vi "Initialise.vi"(8 "error in (no error)":errorcluster, 10 "Message in":refnum<class "InitialiseMessage.lvclass">, 11 "Thorcam in":refnum<class "Thorcam.lvclass">) -> (0 "error out":errorcluster, 3 "Thorcam out":refnum<class "Thorcam.lvclass">)   [LabVIEW 2012, in "Thorcam.lvclass"]
doc: "This method is called when an initialise message is received. It mainly initialises the RabbitMQ connectivity. \n\nOverride this method when your component needs special initialisation (e.g. of software or hardware resources). In that case, don't forget to call the parent for proper implementation. If your component owns subcomponents, they count as resources, so you have to initialise them by calling their own initialise functions"
uses:
  Thorcam.lvclass
  <vilib>/Distrio/Murmex/InitialiseMessage/InitialiseMessage.lvclass
  <vilib>/Distrio/Murmex/Murmex/Murmex.lvclass
  Thorcam.lvclass/Thorcam.ctl
panel:
  # "This method is called when the INTIALISE\ntrigger is sent. \n\nOverride this method when your component needs to\nrespond to this trigger. \n\nCall parent for proper implementation"
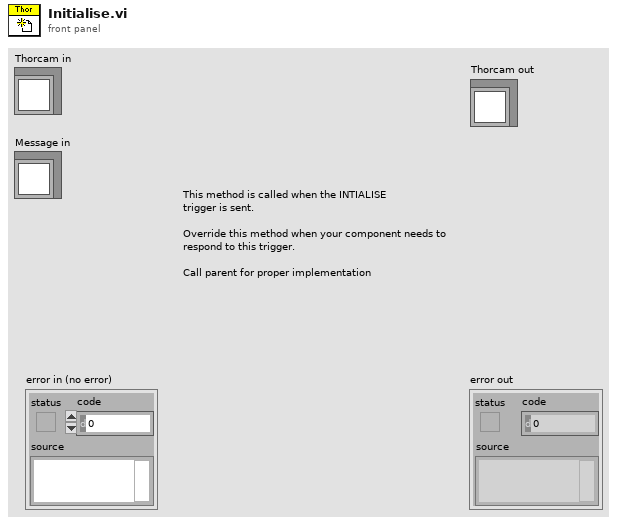
[diagram p1: front panel]
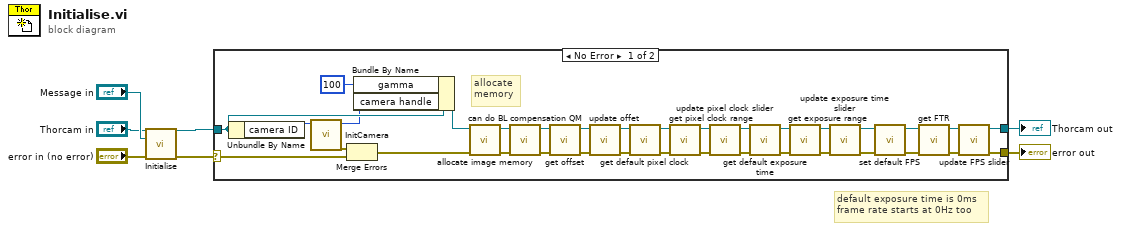
[diagram p0: block diagram]
diagram:
  # "default exposure time is 0ms\nframe rate starts at 0Hz too"
  n1 = call-parent "Initialise.vi"("error in (no error)"="error in (no error)", "Message in"="Message in", "Murmex in"="Thorcam in") -> ("error out"=w4:errorcluster, "Murmex out"=w3:refnum<class "Thorcam.lvclass">)  [unwired: 7 in]
  n2 = case shown="No Error" w4 {
    selector: w4 -> [w41 w42]
    tunnel: w3 -> [w38 w43]
    tunnel: [w27 w42] -> w2
    tunnel: [w28 w43] -> w1
    frame No Error {
      # "allocate\nmemory"
      n3 = Unbundle By Name(w38) -> ("camera ID"=w39:u32)
      n4 = call <instrlib>:"InitCamera.vi"("Camera ID"=w39) -> ("error out"=w40:errorcluster, "Camera Handle Out"=w37:u32)  [unwired: 9 in]
      n5 = Merge Errors(w40, w41) -> (w36:errorcluster)
      n6 = Bundle By Name(cluster=w38, "gamma"=100 ("settings.image.gamma"), "camera handle"=w37) -> (w35:refnum<class "Thorcam.lvclass">)
      n7 = call-dynamic "allocate image memory.vi"("error in (no error)"=w36, "Thorcam in"=w35) -> ("error out"=w34:errorcluster, "Thorcam out"=w33:refnum<class "Thorcam.lvclass">)  [unwired: 8 in]
      n8 = call-dynamic "can do BL compensation QM"("error in (no error)"=w34, "Thorcam in"=w33) -> ("error out"=w31:errorcluster, "Thorcam out"=w32:refnum<class "Thorcam.lvclass">)  [unwired: 8 in]
      n9 = call-dynamic "get offset.vi"("error in (no error)"=w31, "Thorcam in"=w32) -> ("error out"=w30:errorcluster, "Thorcam out"=w29:refnum<class "Thorcam.lvclass">)  [unwired: 8 in]
      n10 = call-dynamic "update offet.vi"("error in (no error)"=w30, "Thorcam in"=w29) -> ("error out"=w15:errorcluster, "Thorcam out"=w16:refnum<class "Thorcam.lvclass">)  [unwired: 8 in]
      n11 = call-dynamic "get default pixel clock.vi"("error in (no error)"=w15, "Thorcam in"=w16) -> ("error out"=w18:errorcluster, "Thorcam out"=w22:refnum<class "Thorcam.lvclass">)  [unwired: 7 in, 1 out]
      n12 = call-dynamic "get pixel clock range.vi"("error in (no error)"=w18, "Thorcam in"=w22) -> ("error out"=w17:errorcluster, "Thorcam out"=w21:refnum<class "Thorcam.lvclass">)  [unwired: 8 in]
      n13 = call-dynamic "update pixel clock slider.vi"("error in (no error)"=w17, "Thorcam in"=w21) -> ("error out"=w13:errorcluster, "Thorcam out"=w14:refnum<class "Thorcam.lvclass">)  [unwired: 8 in]
      n14 = call-dynamic "get default exposure time.vi"("error in (no error)"=w13, "Thorcam in"=w14) -> ("error out"=w20:errorcluster, "Thorcam out"=w24:refnum<class "Thorcam.lvclass">)  [unwired: 7 in, 1 out]
      n15 = call-dynamic "get exposure range.vi"("error in (no error)"=w20, "Thorcam in"=w24) -> ("error out"=w19:errorcluster, "Thorcam out"=w23:refnum<class "Thorcam.lvclass">)  [unwired: 8 in]
      n16 = call-dynamic "update exposure time slider.vi"("error in (no error)"=w19, "Thorcam in"=w23) -> ("error out"=w10:errorcluster, "Thorcam out"=w12:refnum<class "Thorcam.lvclass">)  [unwired: 8 in]
      n17 = call-dynamic "set default FPS.vi"("error in (no error)"=w10, "Thorcam in"=w12) -> ("error out"=w9:errorcluster, "Thorcam out"=w11:refnum<class "Thorcam.lvclass">)  [unwired: 8 in]
      n18 = call-dynamic "get FTR.vi"("error in (no error)"=w9, "Thorcam in"=w11) -> ("error out"=w25:errorcluster, "Thorcam out"=w26:refnum<class "Thorcam.lvclass">)  [unwired: 8 in]
      n19 = call-dynamic "update FPS slider.vi"("error in (no error)"=w25, "Thorcam in"=w26) -> ("error out"=w27:errorcluster, "Thorcam out"=w28:refnum<class "Thorcam.lvclass">)  [unwired: 8 in]
    }
    frame Error {
    }
  }
  "error out" <- w2
  "Thorcam out" <- w1
